vi "Server_Main Data(FGV).vi"(6 "FGV Method(Get)":T1, 8 "error in":errorcluster, 11 "Main Data In":T2) -> (0 "error out":errorcluster, 3 "Main Data Out":T2)   [LabVIEW 2018, in "Cloud Server.lvlib"]
doc: "宣告Server_main.vi常用到參照的暫存記憶體區塊。"
uses:
  Cloud Server.lvlib
  Data Def/Server_Main Data.ctl
  Com VIs/Data Def/stm_MetaElement.ctl
  Com VIs/Data Def/stm_MetaDataElement.ctl
  Data Def/Server_Main Queue.ctl
  Data Def/Server_Server Write Queue Data.ctl
  Data Def/Server_Main Loop Queue Data.ctl
  Data Def/Server_Main Loop State.ctl
  <vilib>/vision/Image Controls.llb/IMAQ Image.ctl
  Data Def/Server_FGV Method.ctl
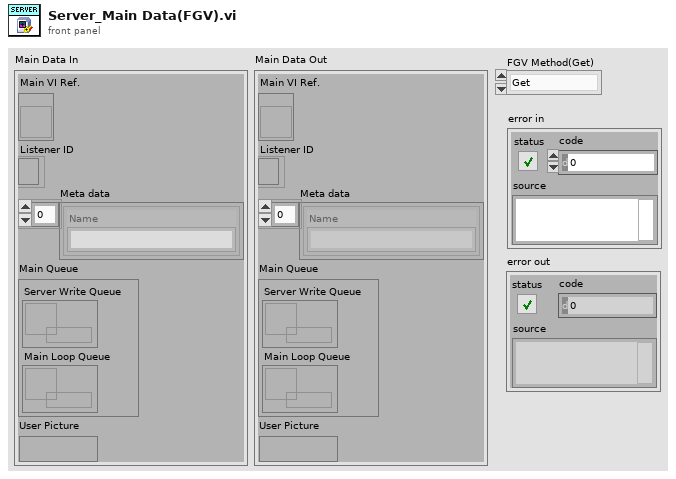
[diagram p1: front panel]
types:
  T1 = typedef "Cloud Server.lvlib/Server_FGV Method.ctl" = enum16{"Get", "Put"}
  T2 = typedef "Cloud Server.lvlib/Server_Main Data.ctl" = cluster{"Main VI Ref.":refnum<vi>, "Listener ID":refnum<k5>, "Meta data":T3[], "Main Queue":T5, "User Picture":T6}
  T3 = typedef "stm_MetaElement.ctl" = cluster{"Name":T4}
  T4 = typedef "stm_MetaDataElement.ctl" = string
  T5 = typedef "Cloud Server.lvlib/Server_Main Queue.ctl" = cluster{"Server Write Queue":refnum<queue>, "Main Loop Queue":refnum<queue>}
  T6 = typedef "IMAQ Image.ctl" = refnum<image>
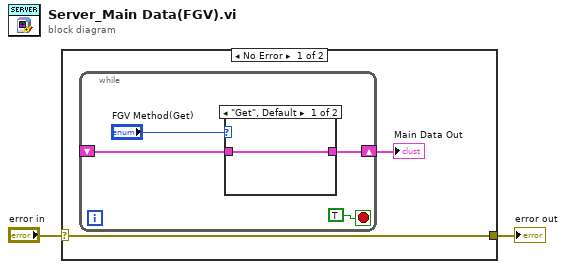
[diagram p0: block diagram]
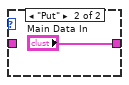
[diagram p2: hidden frame]
diagram:
  n1 = case shown="No Error" "error in" {
    selector: "error in" -> [w3 w11]
    tunnel: [w3 w11] -> w1
    frame No Error {
      n2 = while {
        shift-right: [w6] -> w4
        shift-left: _ -> [w5]
        stop <- TRUE stop-if-true
        n3 = case shown="\"Get\", Default" "FGV Method(Get)" {
          tunnel: [w9 "Main Data In"] -> w6
          tunnel: w5 -> [w9 _]
          frame "Get", Default {
          }
          frame "Put" {
          }
        }
      }
      "Main Data Out" <- w4
    }
    frame Error {
    }
  }
  "error out" <- w1
